vi "FPGA.vi"() -> ()   [LabVIEW 2012]
uses:
  <vilib>/rvi/eio/common/nirviEmuTemplateMethod_errors.vi
  <vilib>/eio/EIONode/EIONode.xnode
panel:
  in  "FPGA LED":bool
  out "Chasis Temp":i16
  in  "Motor5":u16 max=512 step=1
  in  "Motor6":u16 max=512 step=1
  in  "Motor7":u16 max=512 step=1
  in  "Motor8":u16 max=512 step=1
  in  "Motor9":u16 max=512 step=1
  in  "Motor10":u16 max=512 step=1
  in  "Motor11":u16 max=512 step=1
  in  "Motor12":u16 max=512 step=1
  in  "Motor1":u16 max=512 step=1
  in  "Motor2":u16 max=512 step=1
  in  "Motor3":u16 max=512 step=1
  in  "Motor4":u16 max=512 step=1
  in  "Halt Execution":bool
  in  "Dout 1":bool
  in  "Dout 2":bool
  in  "Dout 3":bool
  in  "Dout 4":bool
  in  "Dout 5":bool
  in  "Dout 6":bool
  in  "Dout 7":bool
  in  "Dout 8":bool
  out "Din 1":bool
  out "Din 2":bool
  out "Din 3":bool
  out "Din 4":bool
  out "Din 5":bool
  out "Din 6":bool
  out "Din 7":bool
  out "Din 8":bool
  out "Encoder1":i64
  out "Encoder2":i64
  out "Encoder3":i64
  out "Encoder4":i64
  in  "Reset 1":bool
  in  "Reset 2":bool
  in  "Reset 3":bool
  in  "Reset 4":bool
  in  "Analog 2":fxp<+/-,12,5>
  in  "Analog 4":fxp<+/-,12,5>
  in  "Analog 1":fxp<+/-,12,5>
  in  "Analog 3":fxp<+/-,12,5>
  out "PWM counter":i16
  in  "Stop All Motors":bool
  in  "Status LED":bool
  in  "Emergency Stop":bool
  out "Enc1C":bool
  out "Enc2C":bool
  out "Enc3C":bool
  out "Enc4C":bool
  in  "Cal.1":bool
  in  "Cal.2":bool
  in  "Cal. 3":bool
  in  "Cal. 4":bool
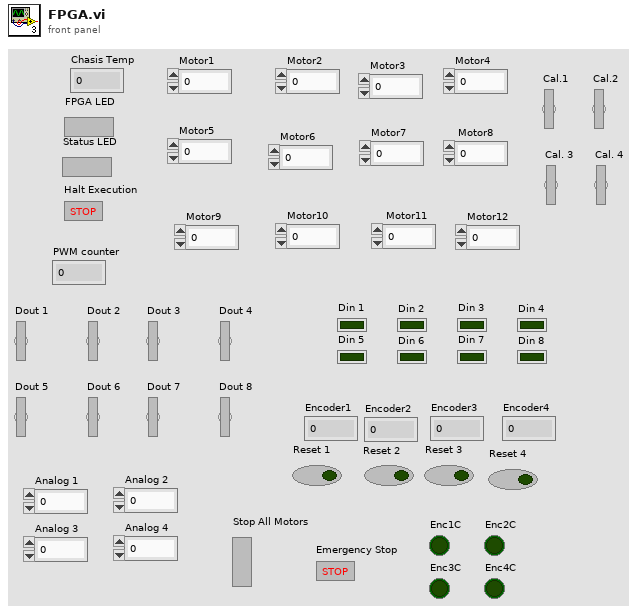
[diagram p1: front panel]
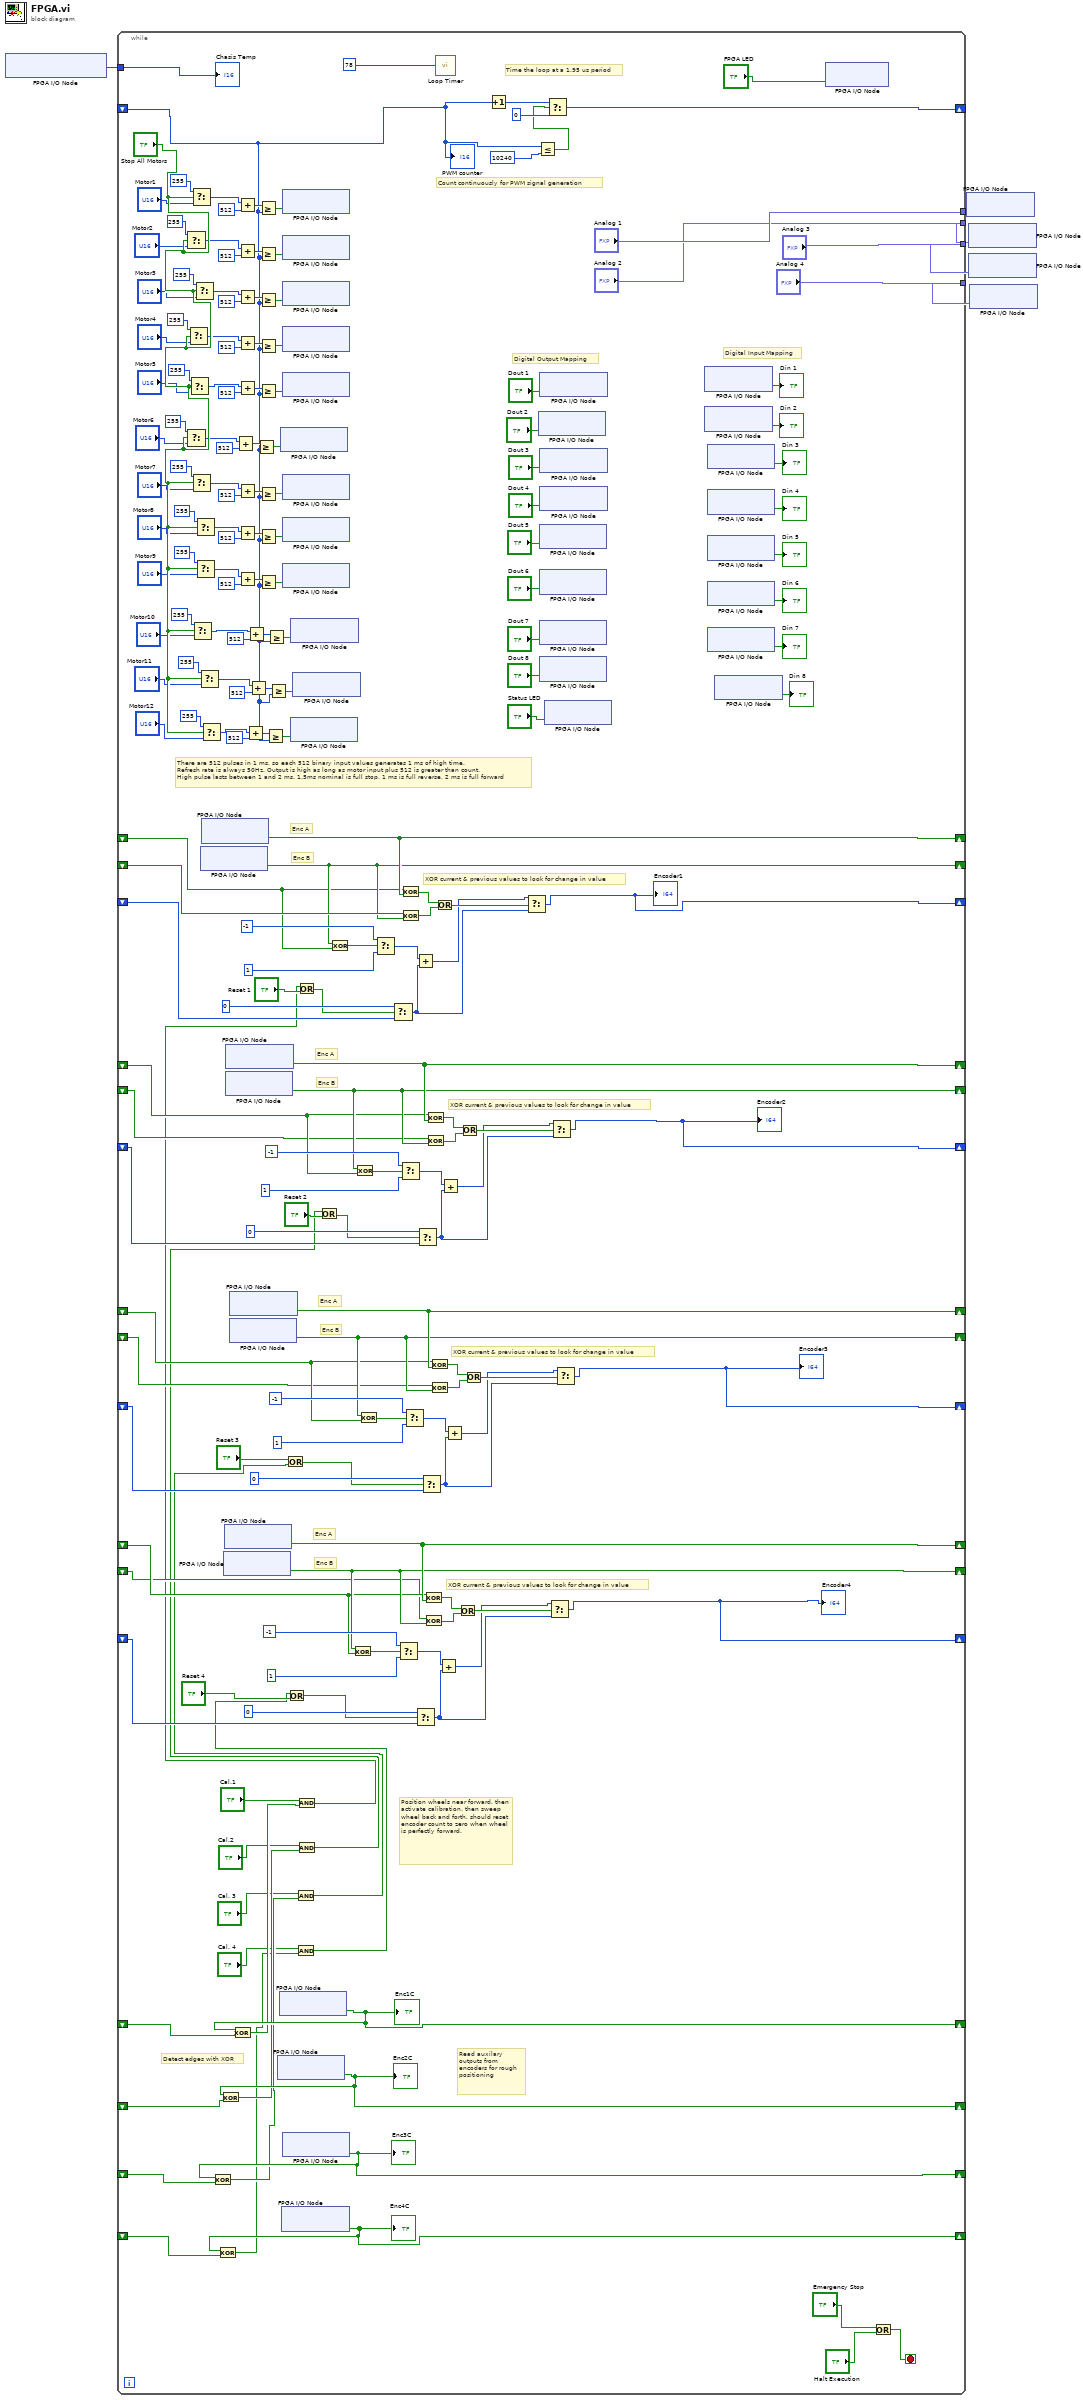
[diagram p0: block diagram]
diagram:
  n1 = xnode "FPGA I/O Node"() -> ("Chassis Temperature"=w5:i16)  [unwired: 1 in, 1 out]
  n2 = while {
    shift-right: [w151] -> _
    shift-left: _ -> [w135]
    shift-right: [w136] -> _
    shift-left: _ -> [w143]
    shift-right: [w145] -> _
    shift-left: _ -> [w144]
    shift-right: [w123] -> _
    shift-left: _ -> [w121]
    shift-right: [w122] -> _
    shift-left: _ -> [w120]
    shift-right: [w119] -> _
    shift-left: _ -> [w118]
    shift-right: [w107] -> _
    shift-left: _ -> [w105]
    shift-right: [w106] -> _
    shift-left: _ -> [w104]
    shift-right: [w102] -> _
    shift-left: _ -> [w103]
    shift-right: [w90] -> _
    shift-left: _ -> [w87]
    shift-right: [w89] -> _
    shift-left: _ -> [w86]
    shift-right: [w88] -> _
    shift-left: _ -> [w85]
    shift-right: [w80] -> _
    shift-left: _ -> [w79]
    tunnel: w5 -> [w77]
    tunnel: ["Analog 1"] -> w4
    tunnel: ["Analog 2"] -> w3
    tunnel: ["Analog 3"] -> w2
    tunnel: ["Analog 4"] -> w1
    shift-right: [w30] -> _
    shift-left: _ -> [w29]
    shift-right: [w28] -> _
    shift-left: _ -> [w27]
    shift-right: [w26] -> _
    shift-left: _ -> [w25]
    shift-right: [w23] -> _
    shift-left: _ -> [w24]
    stop <- w33 stop-if-true
    # "Position wheels near forward, then activate calibration, then sweep wheel back and forth. should reset encoder count to zero when wheel is perfectly forward."
    # "Detect edges with XOR"
    # "Read auxilary outputs from encoders for rough positioning"
    # "Count continuously for PWM signal generation"
    # "Time the loop at a 1.95 us period"
    # "XOR current & previous values to look for change in value"
    # "Enc B"
    # "Enc A"
    # "XOR current & previous values to look for change in value"
    # "Enc B"
    # "Enc A"
    # "XOR current & previous values to look for change in value"
    # "Enc B"
    # "Enc A"
    # "XOR current & previous values to look for change in value"
    # "Enc B"
    # "Enc A"
    # "Digital Input Mapping"
    # "Digital Output Mapping"
    # "There are 512 pulses in 1 ms, so each 512 binary input values generates 1 ms of high time.\nRefresh rate is always 50Hz. Output is high as long as motor input plus 512 is greater than count.\nHigh pulse lasts between 1 and 2 ms. 1.5ms nominal is full stop, 1 ms is full reverse, 2 ms is full forward"
    n3 = Select(t=i16 255, s="Stop All Motors", f="Motor2") -> (s? t:f=w56:u16)
    n4 = Select(t=i16 255, s="Stop All Motors", f="Motor6") -> (s? t:f=w48:u16)
    n5 = Select(t=i16 255, s="Stop All Motors", f="Motor4") -> (s? t:f=w52:u16)
    n6 = Select(t=i16 255, s="Stop All Motors", f="Motor5") -> (s? t:f=w50:u16)
    n7 = Select(t=i16 255, s="Stop All Motors", f="Motor1") -> (s? t:f=w58:u16)
    n8 = Select(t=i16 255, s="Stop All Motors", f="Motor7") -> (s? t:f=w46:u16)
    n9 = Select(t=i16 255, s="Stop All Motors", f="Motor10") -> (s? t:f=w40:u16)
    n10 = Select(t=i16 255, s="Stop All Motors", f="Motor3") -> (s? t:f=w54:u16)
    n11 = Select(t=i16 255, s="Stop All Motors", f="Motor8") -> (s? t:f=w44:u16)
    n12 = Select(t=i16 255, s="Stop All Motors", f="Motor9") -> (s? t:f=w42:u16)
    n13 = Select(t=i16 255, s="Stop All Motors", f="Motor11") -> (s? t:f=w38:u16)
    n14 = xnode "FPGA I/O Node"() -> ("Port7/DIO1"=w136:bool)  [unwired: 1 in, 1 out]
    n15 = xnode "FPGA I/O Node"() -> ("Port7/DIO0"=w151:bool)  [unwired: 1 in, 1 out]
    n16 = Select(t=i16 255, s="Stop All Motors", f="Motor12") -> (s? t:f=w36:u16)
    n17 = xnode "FPGA I/O Node"() -> ("Port4/DIO1"=w89:bool)  [unwired: 1 in, 1 out]
    n18 = xnode "FPGA I/O Node"() -> ("Port4/DIO0"=w90:bool)  [unwired: 1 in, 1 out]
    n19 = xnode "FPGA I/O Node"() -> ("Port3/DIO1"=w122:bool)  [unwired: 1 in, 1 out]
    n20 = xnode "FPGA I/O Node"() -> ("Port3/DIO0"=w123:bool)  [unwired: 1 in, 1 out]
    n21 = xnode "FPGA I/O Node"() -> ("Port3/DIO6"=w106:bool)  [unwired: 1 in, 1 out]
    n22 = xnode "FPGA I/O Node"() -> ("Port3/DIO5"=w107:bool)  [unwired: 1 in, 1 out]
    n23 = Add(x=w48, y=i16 512) -> (x+y=w193:u16)
    n24 = Add(x=w58, y=i16 512) -> (x+y=w203:u16)
    n25 = Add(x=w56, y=i16 512) -> (x+y=w201:u16)
    n26 = Add(x=w54, y=i16 512) -> (x+y=w199:u16)
    n27 = Add(x=w52, y=i16 512) -> (x+y=w197:u16)
    n28 = Add(x=w50, y=i16 512) -> (x+y=w195:u16)
    n29 = Add(x=w46, y=i16 512) -> (x+y=w191:u16)
    n30 = Add(x=w44, y=i16 512) -> (x+y=w189:u16)
    n31 = Add(x=w42, y=i16 512) -> (x+y=w187:u16)
    n32 = Add(x=w36, y=i16 512) -> (x+y=w181:u16)
    n33 = Add(x=w40, y=i16 512) -> (x+y=w185:u16)
    n34 = Add(x=w38, y=i16 512) -> (x+y=w183:u16)
    n35 = Greater Or Equal?(x=w193, y=w79) -> (x >= y?=w174:bool)
    n36 = Greater Or Equal?(x=w203, y=w79) -> (x >= y?=w179:bool)
    n37 = Greater Or Equal?(x=w201, y=w79) -> (x >= y?=w178:bool)
    n38 = Greater Or Equal?(x=w199, y=w79) -> (x >= y?=w177:bool)
    n39 = Greater Or Equal?(x=w197, y=w79) -> (x >= y?=w176:bool)
    n40 = Greater Or Equal?(x=w195, y=w79) -> (x >= y?=w175:bool)
    n41 = Greater Or Equal?(x=w191, y=w79) -> (x >= y?=w173:bool)
    n42 = Greater Or Equal?(x=w189, y=w79) -> (x >= y?=w172:bool)
    n43 = Greater Or Equal?(x=w187, y=w79) -> (x >= y?=w171:bool)
    n44 = Greater Or Equal?(x=w181, y=w79) -> (x >= y?=w168:bool)
    n45 = Greater Or Equal?(x=w185, y=w79) -> (x >= y?=w170:bool)
    n46 = Greater Or Equal?(x=w183, y=w79) -> (x >= y?=w169:bool)
    n47 = xnode "FPGA I/O Node"() -> ("Port3/DIO2"=w28:bool)  [unwired: 1 in, 1 out]
    "Enc2C" <- w28
    n48 = Exclusive Or(1:w27, 2:w28) -> (0:w21:bool)
    n49 = xnode "FPGA I/O Node"() -> ("Port7/DIO2"=w30:bool)  [unwired: 1 in, 1 out]
    "Enc1C" <- w30
    n50 = Exclusive Or(1:w29, 2:w30) -> (0:w22:bool)
    n51 = xnode "FPGA I/O Node"("Port0/DIO5"=w174) -> ()  [unwired: 1 in, 1 out]
    n52 = xnode "FPGA I/O Node"() -> ("Port4/DIO2"=w23:bool)  [unwired: 1 in, 1 out]
    "Enc4C" <- w23
    n53 = Exclusive Or(1:w24, 2:w23) -> (0:w19:bool)
    n54 = xnode "FPGA I/O Node"("Port0/DIO0"=w179) -> ()  [unwired: 1 in, 1 out]
    n55 = xnode "FPGA I/O Node"("Port0/DIO1"=w178) -> ()  [unwired: 1 in, 1 out]
    n56 = xnode "FPGA I/O Node"("Port0/DIO2"=w177) -> ()  [unwired: 1 in, 1 out]
    n57 = xnode "FPGA I/O Node"("Port0/DIO3"=w176) -> ()  [unwired: 1 in, 1 out]
    n58 = xnode "FPGA I/O Node"("Port0/DIO4"=w175) -> ()  [unwired: 1 in, 1 out]
    n59 = xnode "FPGA I/O Node"("Port0/DIO6"=w173) -> ()  [unwired: 1 in, 1 out]
    n60 = xnode "FPGA I/O Node"("Port0/DIO7"=w172) -> ()  [unwired: 1 in, 1 out]
    n61 = xnode "FPGA I/O Node"("Port0/DIO8"=w171) -> ()  [unwired: 1 in, 1 out]
    n62 = xnode "FPGA I/O Node"() -> ("Port3/DIO7"=w26:bool)  [unwired: 1 in, 1 out]
    "Enc3C" <- w26
    n63 = Exclusive Or(1:w25, 2:w26) -> (0:w20:bool)
    n64 = xnode "FPGA I/O Node"("Port1/DIO1"=w168) -> ()  [unwired: 1 in, 1 out]
    n65 = xnode "FPGA I/O Node"("Port1/DIO9"=w170) -> ()  [unwired: 1 in, 1 out]
    n66 = xnode "FPGA I/O Node"("Port1/DIO0"=w169) -> ()  [unwired: 1 in, 1 out]
    n67 = And(x="Cal. 3", y=w20) -> (x .and. y?=w7:bool)
    n68 = Or(x="Reset 3", y=w7) -> (x .or. y?=w12:bool)
    n69 = And(x="Cal. 4", y=w19) -> (x .and. y?=w6:bool)
    n70 = Or(x=w6, y="Reset 4") -> (x .or. y?=w13:bool)
    n71 = And(x="Cal.1", y=w22) -> (x .and. y?=w9:bool)
    n72 = Or(x=w9, y="Reset 1") -> (x .or. y?=w10:bool)
    n73 = And(x="Cal.2", y=w21) -> (x .and. y?=w8:bool)
    n74 = Or(x=w8, y="Reset 2") -> (x .or. y?=w11:bool)
    n75 = Exclusive Or(1:w135, 2:w136) -> (0:w137:bool)
    n76 = Exclusive Or(1:w87, 2:w89) -> (0:w91:bool)
    n77 = Exclusive Or(1:w121, 2:w122) -> (0:w125:bool)
    n78 = Exclusive Or(1:w105, 2:w106) -> (0:w108:bool)
    n79 = Select(t=i16 -1, s=w137, f=i16 1) -> (s? t:f=w139:i16)
    n80 = Select(t=i16 0, s=w10, f=w144) -> (s? t:f=w140:i16)
    n81 = Select(t=i16 -1, s=w91, f=i16 1) -> (s? t:f=w93:i16)
    n82 = Exclusive Or(1:w151, 2:w135) -> (0:w150:bool)
    n83 = Exclusive Or(1:w136, 2:w143) -> (0:w149:bool)
    n84 = Select(t=i16 -1, s=w125, f=i16 1) -> (s? t:f=w127:i16)
    n85 = Select(t=i16 -1, s=w108, f=i16 1) -> (s? t:f=w110:i16)
    n86 = Add(x=w139, y=w140) -> (x+y=w138:i16)
    n87 = Select(t=i16 0, s=w13, f=w85) -> (s? t:f=w94:i16)
    n88 = Select(t=i16 0, s=w11, f=w118) -> (s? t:f=w128:i16)
    n89 = Select(t=i16 0, s=w12, f=w103) -> (s? t:f=w111:i16)
    n90 = Exclusive Or(1:w90, 2:w87) -> (0:w100:bool)
    n91 = Exclusive Or(1:w89, 2:w86) -> (0:w99:bool)
    n92 = Exclusive Or(1:w123, 2:w121) -> (0:w134:bool)
    n93 = Exclusive Or(1:w122, 2:w120) -> (0:w133:bool)
    n94 = Exclusive Or(1:w107, 2:w105) -> (0:w117:bool)
    n95 = Exclusive Or(1:w106, 2:w104) -> (0:w116:bool)
    n96 = Or(x=w150, y=w149) -> (x .or. y?=w148:bool)
    n97 = call "Loop Timer"("Count(Ticks)"=i16 78) -> ()  [unwired: 1 out]
    n98 = Add(x=w93, y=w94) -> (x+y=w92:i16)
    n99 = Add(x=w127, y=w128) -> (x+y=w126:i16)
    n100 = Add(x=w110, y=w111) -> (x+y=w109:i16)
    n101 = Or(x=w100, y=w99) -> (x .or. y?=w98:bool)
    n102 = Or(x=w134, y=w133) -> (x .or. y?=w132:bool)
    n103 = Or(x=w117, y=w116) -> (x .or. y?=w115:bool)
    n104 = Increment(x=w79) -> (x+1=w84:i16)
    n105 = Select(t=w138, s=w148, f=w140) -> (s? t:f=w145:i16)
    "Encoder1" <- w145
    n106 = Less Or Equal?(x=w79, y=i16 10240) -> (x <= y?=w82:bool)
    n107 = xnode "FPGA I/O Node"("Port1/DIO3"="Dout 2") -> ()  [unwired: 1 in, 1 out]
    n108 = xnode "FPGA I/O Node"("Port1/DIO6"="Dout 5") -> ()  [unwired: 1 in, 1 out]
    n109 = xnode "FPGA I/O Node"("Port1/DIO7"="Dout 6") -> ()  [unwired: 1 in, 1 out]
    n110 = xnode "FPGA I/O Node"("Port1/DIO8"="Dout 7") -> ()  [unwired: 1 in, 1 out]
    n111 = xnode "FPGA I/O Node"("Port2/DIO9"="Dout 8") -> ()  [unwired: 1 in, 1 out]
    n112 = xnode "FPGA I/O Node"("Port1/DIO2"="Dout 1") -> ()  [unwired: 1 in, 1 out]
    n113 = xnode "FPGA I/O Node"("Port1/DIO4"="Dout 3") -> ()  [unwired: 1 in, 1 out]
    n114 = xnode "FPGA I/O Node"("Port1/DIO5"="Dout 4") -> ()  [unwired: 1 in, 1 out]
    n115 = xnode "FPGA I/O Node"("Port2/DIO1"="Status LED") -> ()  [unwired: 1 in, 1 out]
    n116 = Select(t=w84, s=w82, f=i16 0) -> (s? t:f=w80:i16)
    n117 = Select(t=w92, s=w98, f=w94) -> (s? t:f=w88:i16)
    "Encoder4" <- w88
    n118 = Select(t=w126, s=w132, f=w128) -> (s? t:f=w119:i16)
    "Encoder2" <- w119
    n119 = Select(t=w109, s=w115, f=w111) -> (s? t:f=w102:i16)
    "Encoder3" <- w102
    n120 = xnode "FPGA I/O Node"() -> ("Port3/DIO8"=→"Din 1":bool)  [unwired: 1 in, 1 out]
    n121 = xnode "FPGA I/O Node"() -> ("Port4/DIO9"=→"Din 2":bool)  [unwired: 1 in, 1 out]
    n122 = xnode "FPGA I/O Node"() -> ("Port4/DIO3"=→"Din 3":bool)  [unwired: 1 in, 1 out]
    n123 = xnode "FPGA I/O Node"() -> ("Port4/DIO4"=→"Din 4":bool)  [unwired: 1 in, 1 out]
    n124 = xnode "FPGA I/O Node"() -> ("Port4/DIO5"=→"Din 5":bool)  [unwired: 1 in, 1 out]
    n125 = xnode "FPGA I/O Node"() -> ("Port4/DIO6"=→"Din 6":bool)  [unwired: 1 in, 1 out]
    n126 = xnode "FPGA I/O Node"() -> ("Port4/DIO7"=→"Din 7":bool)  [unwired: 1 in, 1 out]
    n127 = xnode "FPGA I/O Node"() -> ("Port4/DIO8"=→"Din 8":bool)  [unwired: 1 in, 1 out]
    n128 = xnode "FPGA I/O Node"("FPGA LED"="FPGA LED") -> ()  [unwired: 1 in, 1 out]
    n129 = Or(x="Emergency Stop", y="Halt Execution") -> (x .or. y?=w33:bool)
    "Chasis Temp" <- w77
    "PWM counter" <- w79
  }
  n130 = xnode "FPGA I/O Node"("ModB/AO0"=w4) -> ()  [unwired: 1 in, 1 out]
  n131 = xnode "FPGA I/O Node"("ModB/AO1"=w3) -> ()  [unwired: 1 in, 1 out]
  n132 = xnode "FPGA I/O Node"("ModB/AO2"=w2) -> ()  [unwired: 1 in, 1 out]
  n133 = xnode "FPGA I/O Node"("ModB/AO3"=w1) -> ()  [unwired: 1 in, 1 out]
